vi "GenerateTableNames.vi"(8 "error in (no error)":errorcluster, 10 "Path":path, 11 "ReportList in":refnum<class "ReportList.lvclass">) -> (0 "error out":errorcluster, 3 "ReportList out":refnum<class "ReportList.lvclass">)   [LabVIEW 2015, in "ReportList.lvclass"]
uses:
  ReportList.lvclass
  _list/List.lvclass/List.ctl
  <vilib>/Utility/file.llb/Read Delimited Spreadsheet (string).vi
  _list/List.lvclass
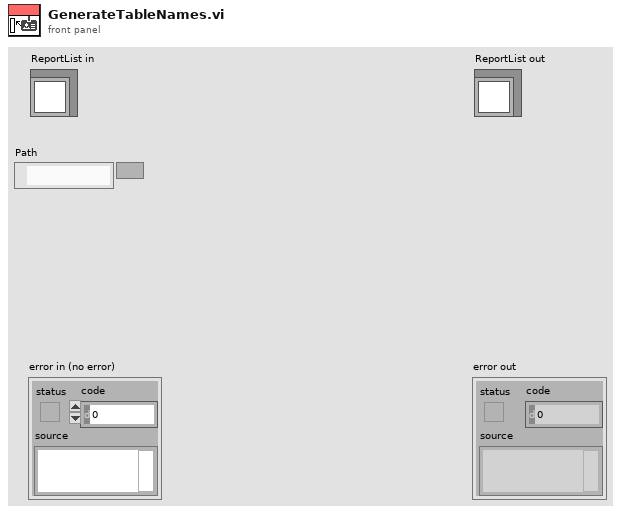
[diagram p1: front panel]
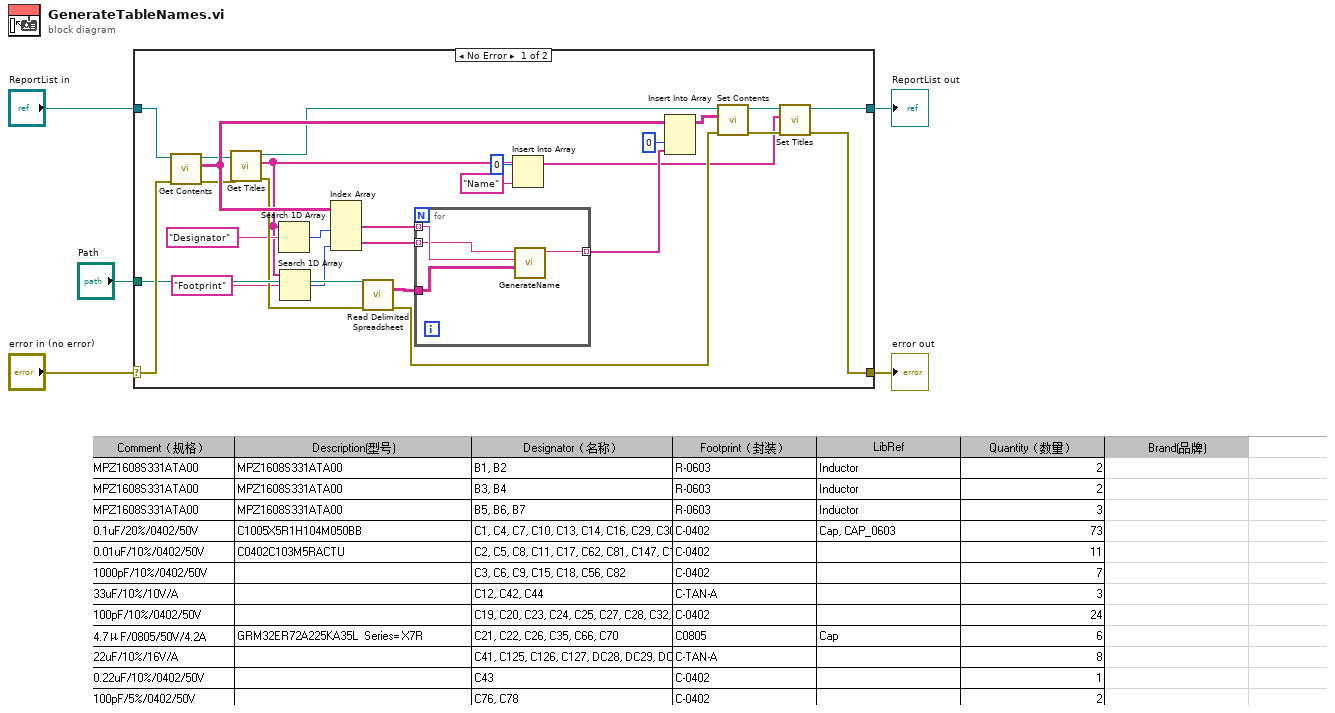
[diagram p0: block diagram]
diagram:
  n1 = case shown="No Error" "error in (no error)" {
    selector: "error in (no error)" -> [w31 w38]
    tunnel: [w14 w38] -> w4
    tunnel: [w15 w37] -> w2
    tunnel: "ReportList in" -> [w32 w37]
    tunnel: "Path" -> [w28 _]
    frame No Error {
      n2 = call "Get Contents.vi"("error in (no error)"=w31, "List in"=w32) -> ("error out"=w20:errorcluster, "Contents"=w26:string[][], "List out"=w21:refnum<class "ReportList.lvclass">)  [unwired: 7 in]
      n3 = call "Get Titles.vi"("error in (no error)"=w20, "List in"=w21) -> ("error out"=w19:errorcluster, "Titles"=w9:string[], "List out"=w18:refnum<class "ReportList.lvclass">)  [unwired: 7 in]
      n4 = Search 1D Array(1D array=w9, element="Designator") -> (index of element=w7:i32)  [unwired: 1 in]
      n5 = Search 1D Array(1D array=w9, element="Footprint") -> (index of element=w6:i32)  [unwired: 1 in]
      n6 = Index Array(array=w26, index (col) #1=w7, index (col) #2=w6) -> (element #1=w30:string[], element #2=w29:string[])  [unwired: 2 in]
      n7 = call-poly <vilib>:"Read Delimited Spreadsheet.vi"("file path (dialog if empty)"=w28, "error in (no error)"=w19) -> ("all rows"=w27:string[][], "error out"=w22:errorcluster)  [unwired: 8 in, 4 out]
      n8 = for {
        tunnel: w30 -> [w36] mode=indexing
        tunnel: w29 -> [w35] mode=indexing
        tunnel: [w34] -> w24 mode=indexing
        tunnel: w27 -> [w33]
        n9 = call "GenerateName.vi"("Rules"=w33, "Designator"=w36, "Footprint"=w35) -> ("Name"=w34:string)  [unwired: 8 in]
      }
      n10 = Insert Into Array(array=w9, index=0, new element="Name" ("new element/subarray")) -> (w12:string[])
      n11 = Insert Into Array(array=w26, index (col)=0 ("disabled index (col)"), new element=w24) -> (w23:string[][])  [unwired: 1 in]
      n12 = call "Set Contents.vi"("error in (no error)"=w22, "Contents"=w23, "List in"=w18) -> ("error out"=w16:errorcluster, "List out"=w17:refnum<class "ReportList.lvclass">)  [unwired: 7 in]
      n13 = call "Set Titles.vi"("error in (no error)"=w16, "Titles"=w12, "List in"=w17) -> ("error out"=w14:errorcluster, "List out"=w15:refnum<class "ReportList.lvclass">)  [unwired: 7 in]
    }
    frame Error {
    }
  }
  "error out" <- w4
  "ReportList out" <- w2
